vi "LaunchPad Receive Loop.vi"(10 "Telemetry Notifier Ref":refnum<notifier>, 11 "Telemetry Queue Ref":refnum<queue>) -> ()   [LabVIEW 2015]
uses:
  Telemetry Packet Type.ctl
  Thermocouple Data.ctl
panel:
  out "Packet Count":u32
  out "Error Count":u32
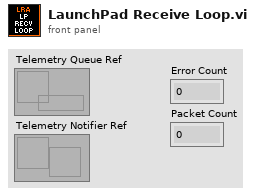
[diagram p1: front panel]
types:
  T1 = typedef "Telemetry Packet Type.ctl" = cluster{"Timestamp\n":u32, "Transducer Value":u16[], "Main Loop Rate":u32, "Solenoid State":bool[], "Output Enabled":bool, "Solenoids Powered":bool, "TC Data":T2[], "TD Rate":u32, "TD Execution Time":u32, "TC Rate":u32, "TC Execution Time":u32}
  T2 = typedef "Thermocouple Data.ctl" = cluster{"TC Temp":dbl, "Internal Temp":dbl, "Fault":bool, "Short to VCC":bool, "Short to GND":bool, "Open Circuit":bool}
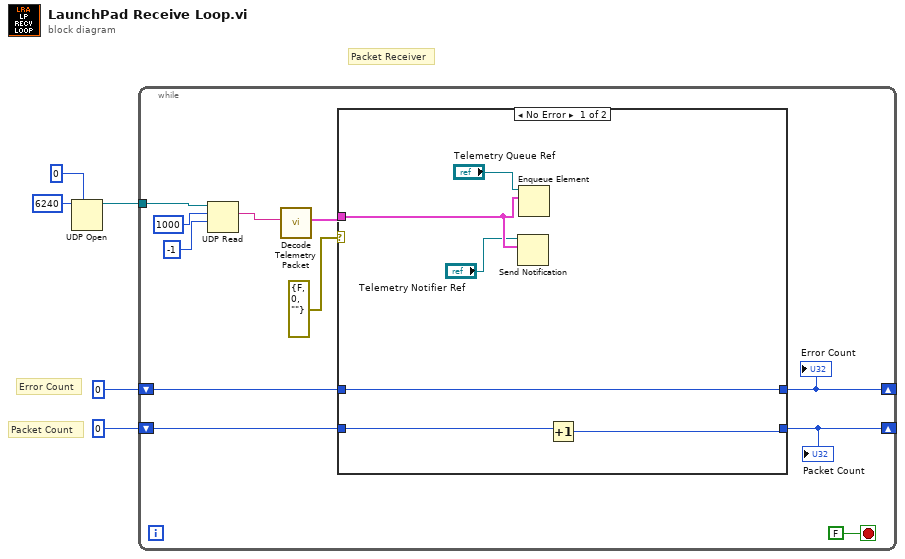
[diagram p0: block diagram]
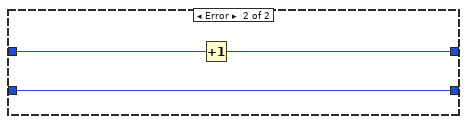
[diagram p2: hidden frame]
diagram:
  # "Packet Receiver"
  # "Packet Count"
  # "Error Count"
  n1 = UDP Open(7:u32 0 ("net address"), 11:u16 6240 ("port")) -> (port=w4:refnum<k16>)  [unwired: 3 in, 2 out]
  n2 = while {
    tunnel: w4 -> [w15]
    shift-right: [w11] -> _
    shift-left: u32 0 ("net address") -> [w12]
    shift-right: [w10] -> _
    shift-left: u32 0 ("net address") -> [w9]
    stop <- FALSE stop-if-true
    n3 = UDP Read(connection ID=w15, max size (548)=1000, timeout ms (25000)=-1) -> (data out=w8:string)  [unwired: 1 in, 4 out]
    n4 = call "Decode Telemetry Packet.vi"("Packet Data String"=w8) -> ("Telemetry Packet"=w7:T1)  [unwired: 10 in]
    n5 = case shown="No Error" errorcluster {"status"=FALSE, "code"=0, "source"=""} ("error IO") {
      tunnel: w7 -> [w21 _]
      tunnel: w12 -> [w19 w25]
      tunnel: [w19 w24] -> w11
      tunnel: [w17 w23] -> w10
      tunnel: w9 -> [w18 w23]
      frame No Error {
        n6 = Send Notification(notification=w21, notifier="Telemetry Notifier Ref") -> ()  [unwired: 1 in, 2 out]
        n7 = Enqueue Element(queue="Telemetry Queue Ref", element=w21) -> ()  [unwired: 2 in, 3 out]
        n8 = Increment(x=w18) -> (x+1=w17:u32)
      }
      frame Error {
        n9 = Increment(x=w25) -> (x+1=w24:u32)
      }
    }
    "Error Count" <- w11
    "Packet Count" <- w10
  }
